vi "Configure Parameter 1.vi"(8 "error in (no error)":errorcluster, 10 "value":u16, 11 "PLBB in":refnum<class "Test Device.lvclass">) -> (0 "error out":errorcluster, 3 "PLBB out":refnum<class "Test Device.lvclass">)   [LabVIEW 2015, in "Test Device.lvclass"]
uses:
  Test Device.lvclass
  <vilib>/plasmapper/PL Modbus Client/PL Modbus Client.lvclass
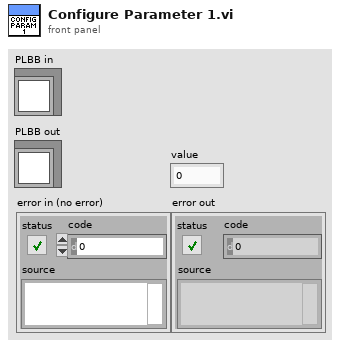
[diagram p1: front panel]
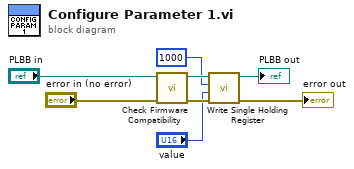
[diagram p0: block diagram]
diagram:
  n1 = call-dynamic "Check Firmware Compatibility.vi"("error in (no error)"="error in (no error)", "TD in"="PLBB in") -> ("error out"=w6:errorcluster, "TD out"=w5:refnum<class "Test Device.lvclass">)  [unwired: 8 in]
  n2 = call <vilib>:"Write Single Holding Register.vi"("error in (no error)"=w6, "value"="value", "address"=u16 1000, "MODBUS in"=w5) -> ("error out"=→"error out":errorcluster, "MODBUS out"=→"PLBB out":refnum<class "Test Device.lvclass">)  [unwired: 6 in]
